vi "NavX.vi"(0 "PID gains":T1={"proportional gain (Kc)"=1.0, "integral time (Ti, min)"=0.01, "derivative time (Td, min)"=0.0} {"derivative time (Td, min)" format="%.3f"; "integral time (Ti, min)" format="%.3f"; "proportional gain (Kc)" format="%.3f"}, 1 "AngleSetpoint":dbl, 2 "MaxSpeed":dbl, 3 "NavxSpeed":dbl, 4 "NavX_P":dbl=0.1, 5 "PID?":bool) -> (6 "LeftNavx":dbl, 7 "RightNavx":dbl, 8 "Done?":bool)   [LabVIEW 2017]
uses:
  Robot Global Data.vi
  <vilib>/addons/control/pid/pid.llb/PID (DBL).vi
  <vilib>/addons/control/pid/NI_PID_pid.lvlib
panel:
  in  "Deadband Velocity":dbl=1.0
  in  "Deadband Pos":dbl=1.0
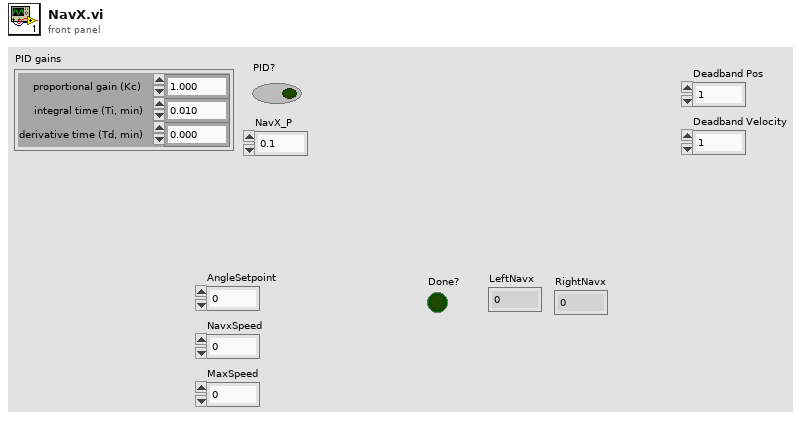
[diagram p1: front panel]
types:
  T1 = cluster{"proportional gain (Kc)":dbl, "integral time (Ti, min)":dbl, "derivative time (Td, min)":dbl}
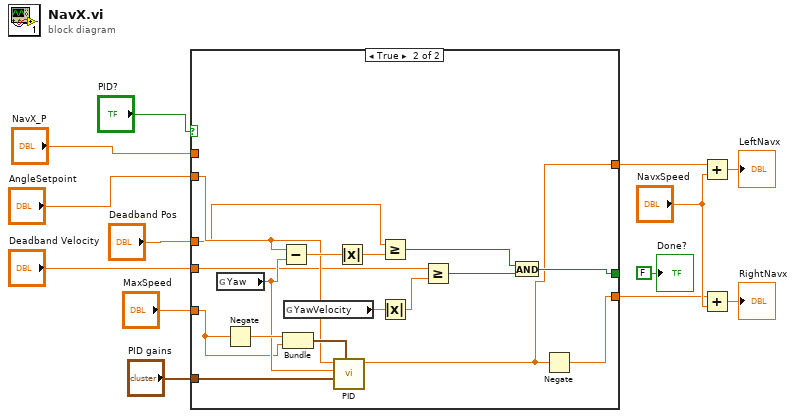
[diagram p0: block diagram]
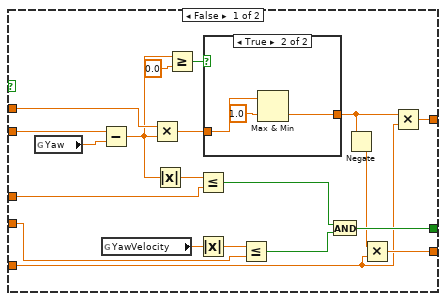
[diagram p2: hidden frame]
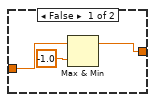
[diagram p3: hidden frame]
diagram:
  n1 = case shown="True" "PID?" {
    tunnel: "AngleSetpoint" -> [w19 w50]
    tunnel: "PID gains" -> [_ w56]
    tunnel: [w20 w43] -> _
    tunnel: "NavX_P" -> [w32 _]
    tunnel: "Deadband Pos" -> [w23 w49]
    tunnel: "Deadband Velocity" -> [w24 w46]
    tunnel: "MaxSpeed" -> [w16 w42]
    tunnel: [w18 w41] -> w4
    tunnel: [w17 w40] -> w2
    frame False {
      n2 = global read "Robot Global Data.vi" "Yaw"() -> (w33:dbl)
      n3 = Subtract(x=w19, y=w33) -> (x-y=w28:dbl)
      n4 = global read "Robot Global Data.vi" "YawVelocity"() -> (w26:dbl)
      n5 = Multiply(x=w32, y=w28) -> (x*y=w29:dbl)
      n6 = Absolute Value(x=w28) -> (abs(x)=w27:dbl)
      n7 = Greater Or Equal?(x=w28, y=0.0) -> (x >= y?=w30:bool)
      n8 = Less Or Equal?(x=w27, y=w23) -> (x <= y?=w21:bool)
      n9 = Absolute Value(x=w26) -> (abs(x)=w25:dbl)
      n10 = case shown="True" w30 {
        tunnel: w29 -> [w36 w39]
        tunnel: [w34 w37] -> w15
        frame False {
          n11 = Max & Min(x=w36, y=-1.0) -> (max(x,y)=w34:dbl)  [unwired: 1 out]
        }
        frame True {
          n12 = Max & Min(x=w39, y=1.0) -> (min(x,y)=w37:dbl)  [unwired: 1 out]
        }
      }
      n13 = Less Or Equal?(x=w25, y=w24) -> (x <= y?=w22:bool)
      n14 = And(x=w21, y=w22) -> (x .and. y?=w20:bool)
      n15 = Negate(x=w15) -> (-x=w14:dbl)
      n16 = Multiply(x=w14, y=w16) -> (x*y=w17:dbl)
      n17 = Multiply(x=w15, y=w16) -> (x*y=w18:dbl)
    }
    frame True {
      n18 = global read "Robot Global Data.vi" "Yaw"() -> (w51:dbl)
      n19 = Negate(x=w42) -> (-x=w55:dbl)
      n20 = Subtract(x=w50, y=w51) -> (x-y=w52:dbl)
      n21 = Bundle(w55, "MaxSpeed"=w42) -> (w54:cluster{dbl, "MaxSpeed":dbl})  [unwired: 1 in]
      n22 = global read "Robot Global Data.vi" "YawVelocity"() -> (w47:dbl)
      n23 = call-poly <vilib>:"PID.vi"("output range"=w54, "PID gains"=w56, "process variable"=w51, "setpoint"=w50) -> ("output"=w41:dbl)  [unwired: 6 in, 1 out]
      n24 = Absolute Value(x=w52) -> (abs(x)=w53:dbl)
      n25 = Greater Or Equal?(x=w49, y=w53) -> (x >= y?=w45:bool)
      n26 = Absolute Value(x=w47) -> (abs(x)=w48:dbl)
      n27 = Greater Or Equal?(x=w46, y=w48) -> (x >= y?=w44:bool)
      n28 = And(x=w45, y=w44) -> (x .and. y?=w43:bool)
      n29 = Negate(x=w41) -> (-x=w40:dbl)
    }
  }
  n30 = Add(x=w4, y="NavxSpeed") -> (x+y=→"LeftNavx":dbl)
  n31 = Add(x=w2, y="NavxSpeed") -> (x+y=→"RightNavx":dbl)
  "Done?" <- FALSE
